vi "bang_bang_controller_FlywheelSim_example.vi"() -> ()   [LabVIEW 2019]
uses:
  <vilib>/Rock Robotics/WPI/ThirdParty/JAS_Junk/TrajLib/BangBang_AtSetpoint.vi
  <vilib>/Rock Robotics/WPI/ThirdParty/JAS_Junk/TrajLib/BangBang_New.vi
  <vilib>/Rock Robotics/WPI/ThirdParty/JAS_Junk/TrajLib/BangBang_Calculate_SP_PV.vi
  <vilib>/Rock Robotics/WPI/ThirdParty/JAS_Junk/TrajLib/Trajectory_Library.lvlib
panel:
  in  "Tab Control":enum32{"Control"}(tab)
  in  "GO DOWN":bool
  out "Battery Voltage":dbl format="%20.3f"
  out "CO Chart":cluster{dbl, "Voltage":dbl}(graph)
  in  "GO UP":bool
  out "Elevator\nHeight \nSetpoint(SP)":dbl(slide) scale=-1.0..6.0
  out "Elevator\nHeight (PV)":dbl(slide) scale=-1.0..6.0
  out "PV Chart":T1(graph)
  out "Motor Dmd (CO)":dbl format="%20.3f"
  out "Top":bool
  out "Bottom":bool
  out "Motor Amps":dbl format="%20.3f"
  # "Bang Bang Control of a simulated elevator"
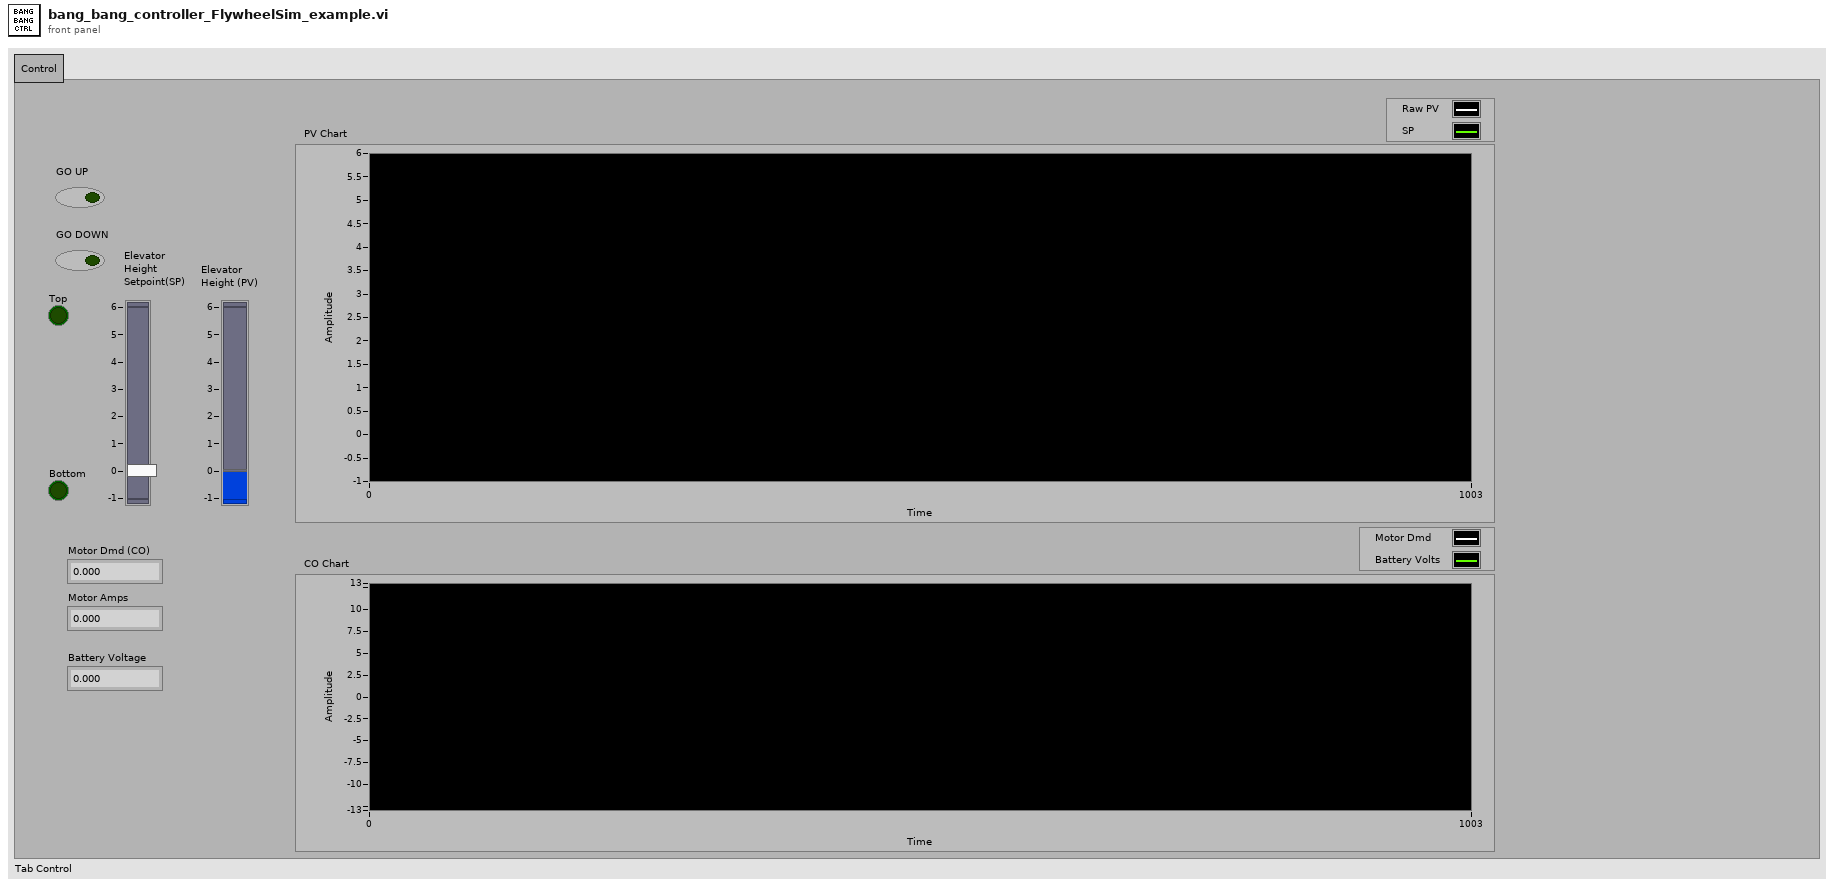
[diagram p1: front panel]
types:
  T1 = cluster{"Position_Meters":dbl, "Real Matrix Element":dbl}
  T2 = typedef "Trajectory_Library.lvlib/ELEVATOR_SIM.ctl" = cluster{"LinearSystemSim":T3, "GearBox":T6, "Gearing":dbl, "DrumRadius_M":dbl, "MinHeight_M":dbl, "MaxHeight_M":dbl, "CarriageMass_Kg":dbl, "SimulateGravity":bool}
  T3 = typedef "Trajectory_Library.lvlib/LINEAR_SYSTEM_SIM.ctl" = cluster{"m_Plant":T4, "m_X":T5, "m_Y":T5, "m_U":T5, "MeasureStdDev":T5}
  T4 = typedef "Trajectory_Library.lvlib/LINEAR_SYSTEM.ctl" = cluster{"m_A":T5, "m_B":T5, "m_C":T5, "m_D":T5, "States":i32, "Inputs":i32, "Outputs":i32}
  T5 = typedef "NI_Matrix.lvlib/RealMatrix.ctl" = dbl[][]
  T6 = typedef "Trajectory_Library.lvlib/DCMOTOR.CTL" = cluster{"nominalVoltage_Volts":dbl, "StallTorque_NM":dbl, "StallCurrent_Amps":dbl, "FreeCurrent_Amps":dbl, "FreeSpeed_RadPerSec":dbl, "R_Ohms":dbl, "KvINV_RadPerSecPerVolt":dbl, "Kt_NMPerAmp":dbl, "L_H":dbl, "Jr_KgM2":dbl}
  T7 = cluster{"ControlOutput":dbl, "Loaded Voltage":dbl}
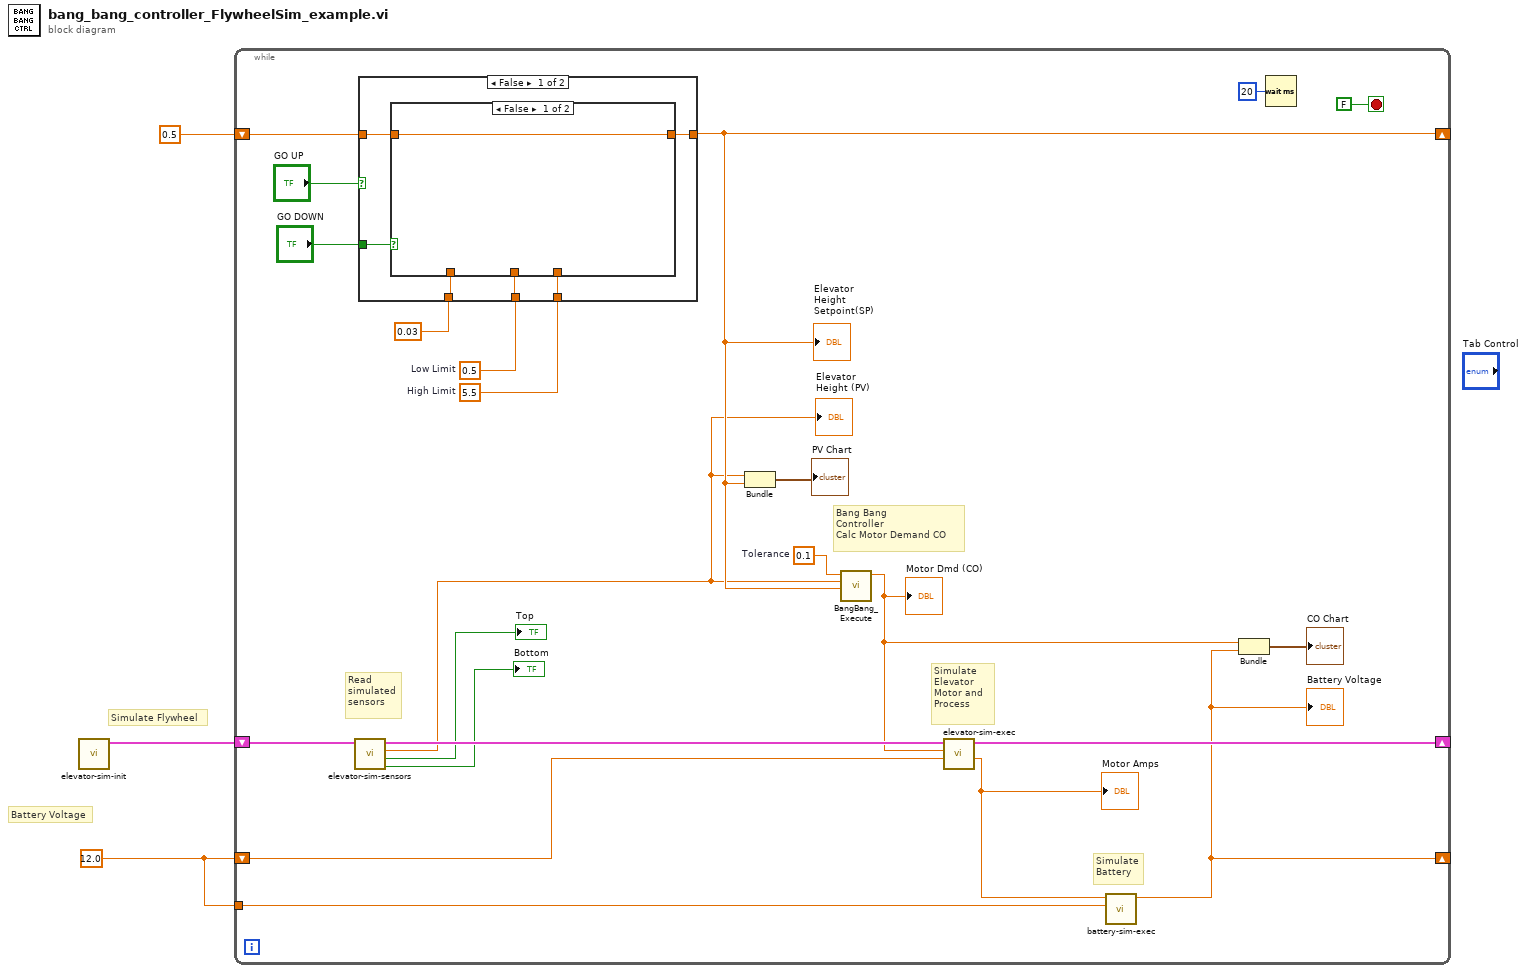
[diagram p0: block diagram]
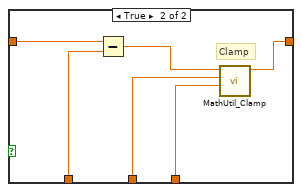
[diagram p2: hidden frame]
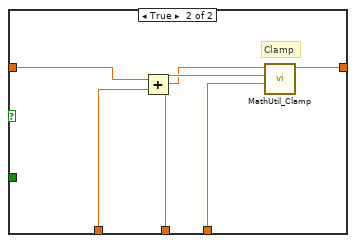
[diagram p3: hidden frame]
diagram:
  w3 = 12.0
  # "Simulate Flywheel"
  # "Battery Voltage"
  n1 = call "elevator-sim-init.vi"() -> ("ElevatorSim"=w2:T2)  [unwired: 11 in]
  n2 = while {
    shift-right: [w22] -> _
    shift-left: w2 -> [w13]
    shift-right: [w8] -> _
    shift-left: w3 -> [w6]
    tunnel: w3 -> [w5]
    shift-right: [w14] -> _
    shift-left: 0.5 -> [w17]
    stop <- FALSE stop-if-true
    w19 = 5.5  # High Limit
    w18 = 0.5  # Low Limit
    w21 = 0.1  # Tolerance
    # "Simulate\nBattery"
    # "Simulate \nElevator\nMotor and \nProcess"
    # "Bang Bang\nController\nCalc Motor Demand CO"
    # "Read\nsimulated\nsensors"
    n3 = call "elevator-sim-sensors.vi"("inElevatorSim"=w13) -> ("AtLowLimit"=→"Bottom":bool, "At HIgh LImit"=→"Top":bool, "Height"=w11:dbl, "outElevatorSim"=w12:T2)  [unwired: 7 in]
    "Elevator\nHeight (PV)" <- w11
    n4 = case shown="False" "GO UP" {
      tunnel: w19 -> [w32 w45]
      tunnel: w18 -> [w31 w44]
      tunnel: w17 -> [w30 w41]
      tunnel: [w29 w43] -> w14
      tunnel: 0.03 ("y") -> [w28 w40]
      tunnel: "GO DOWN" -> [w27 _]
      frame False {
        n5 = case shown="False" w27 {
          tunnel: w32 -> [_ w38]
          tunnel: w31 -> [_ w37]
          tunnel: w30 -> [w33 w36]
          tunnel: [w33 w35] -> w29
          tunnel: w28 -> [_ w34]
          frame False {
          }
          frame True {
            # "Clamp"
            n6 = Subtract(x=w36, y=w34) -> (x-y=w39:dbl)
            n7 = call <vilib>:"MathUtil_Clamp.vi"("High Limit"=w38, "Low Limit"=w37, "Value"=w39) -> ("Result"=w35:dbl)  [unwired: 8 in]
          }
        }
      }
      frame True {
        # "Clamp"
        n8 = Add(x=w41, y=w40) -> (x+y=w42:dbl)
        n9 = call <vilib>:"MathUtil_Clamp.vi"("High Limit"=w45, "Low Limit"=w44, "Value"=w42) -> ("Result"=w43:dbl)  [unwired: 8 in]
      }
    }
    "Elevator\nHeight \nSetpoint(SP)" <- w14
    n10 = Bundle("Height"=w11, "Result"=w14) -> (→"PV Chart":cluster{"Height":dbl, "Result":dbl})  [unwired: 1 in]
    n11 = call <vilib>:"BangBang_Execute.vi"("Setpoint"=w14, "Measurment"=w11, "Tolerance"=w21) -> ("ControlOutput"=w4:dbl)  [unwired: 6 in, 2 out]
    "Motor Dmd (CO)" <- w4
    n12 = call "elevator-sim-exec.vi"("Battery Voltage"=w6, "Motor Dmd CO"=w4, "inElevatorSim"=w12) -> ("Current"=w7:dbl, "out ElevatorSim"=w22:T2)  [unwired: 7 in]
    "Motor Amps" <- w7
    n13 = call "battery-sim-exec.vi"("Nominal Battery\nVoltage"=w5, "Current Amps"=w7) -> ("Loaded Voltage"=w8:dbl)  [unwired: 9 in]
    "Battery Voltage" <- w8
    n14 = Bundle("ControlOutput"=w4, "Loaded Voltage"=w8) -> (→"CO Chart":T7)  [unwired: 1 in]
    n15 = Wait (ms)(milliseconds to wait=u32 20) -> ()  [unwired: 1 out]
  }
